vi "Auto-Refresh Start.vi"(8 "error in (no error)":errorcluster, 11 "SimSyA in":refnum<class "SimSyA.lvclass">) -> (0 "error out":errorcluster, 3 "SimSyA out":refnum<class "SimSyA.lvclass">)   [LabVIEW 2014, in "SimSyA.lvlib" / "SimSyA.lvclass"]
uses:
  SimSyA.lvclass
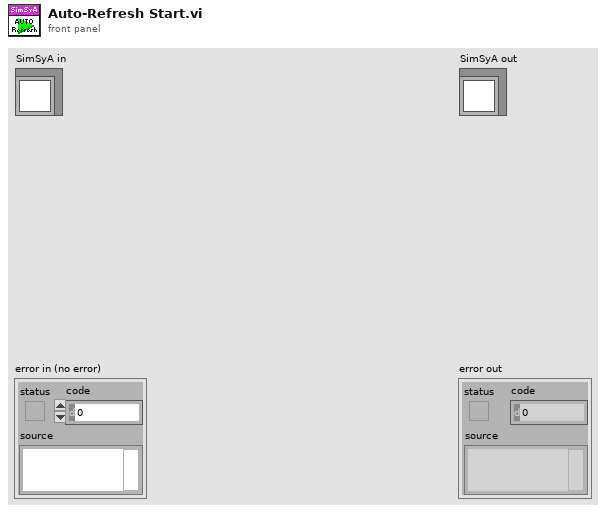
[diagram p1: front panel]
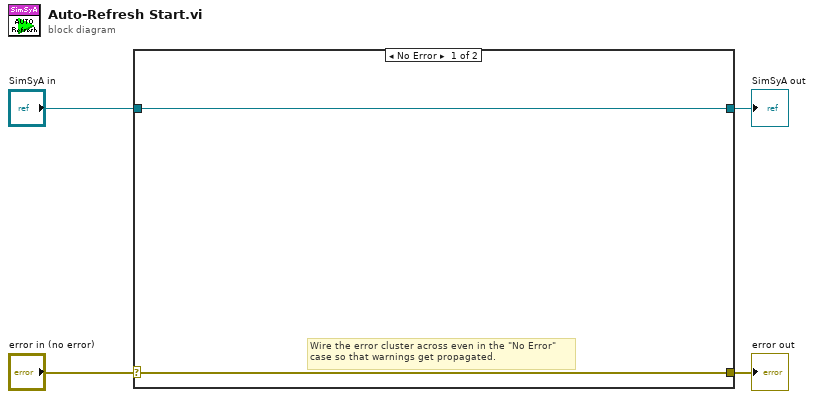
[diagram p0: block diagram]
diagram:
  n1 = case shown="No Error" "error in (no error)" {
    selector: "error in (no error)" -> [w5 w8]
    tunnel: [w5 w8] -> w3
    tunnel: [w6 w7] -> w1
    tunnel: "SimSyA in" -> [w6 w7]
    frame No Error {
      # "Wire the error cluster across even in the \"No Error\"\ncase so that warnings get propagated."
    }
    frame Error {
    }
  }
  "error out" <- w3
  "SimSyA out" <- w1
